vi "Init Airmar Serial.vi"(8 "error in (no error)":errorcluster, 10 "NotifierReff":T1, 11 "VISA Refnum in":refnum<visa-resource-name>="COM1") -> (0 "error out":errorcluster, 2 "Total number of connection attempts":i32, 3 "VISA Refnum out":refnum<visa-resource-name>)   [LabVIEW 2013]
doc: "This VI checks to see if the sensor is communicating on 4800 or 38400 baud and sets it to 38400 baud if it is not already."
uses:
  Data/TypeDefs/Notifiers.ctl
  Data/TypeDefs/UTM Location.ctl
  Data/TypeDefs/Sail Set Suggestions.ctl
  Data/TypeDefs/Rudder Set Suggestions.ctl
  Data/TypeDefs/OverrideInformation.ctl
  Data/TypeDefs/OverrideMode.ctl
  Data/TypeDefs/MotorSetup.ctl
  Data/TypeDefs/DynamixelSetupInfo.ctl
  Data/TypeDefs/AirmarStatus.ctl
  Data/TypeDefs/HardwareOnline.ctl
  Data/TypeDefs/DynamixelCycleTracker.ctl
  Data/TypeDefs/RC Input Values.ctl
  Classes/Waypoint/Waypoint.lvclass
panel:
  out "return count":u32
  out "read buffer 3":string
  out "read buffer 2":string
  out "read buffer":string
  out "# of 38400 baud attempts":i32
  out "# of 4800 baud attempts":i32
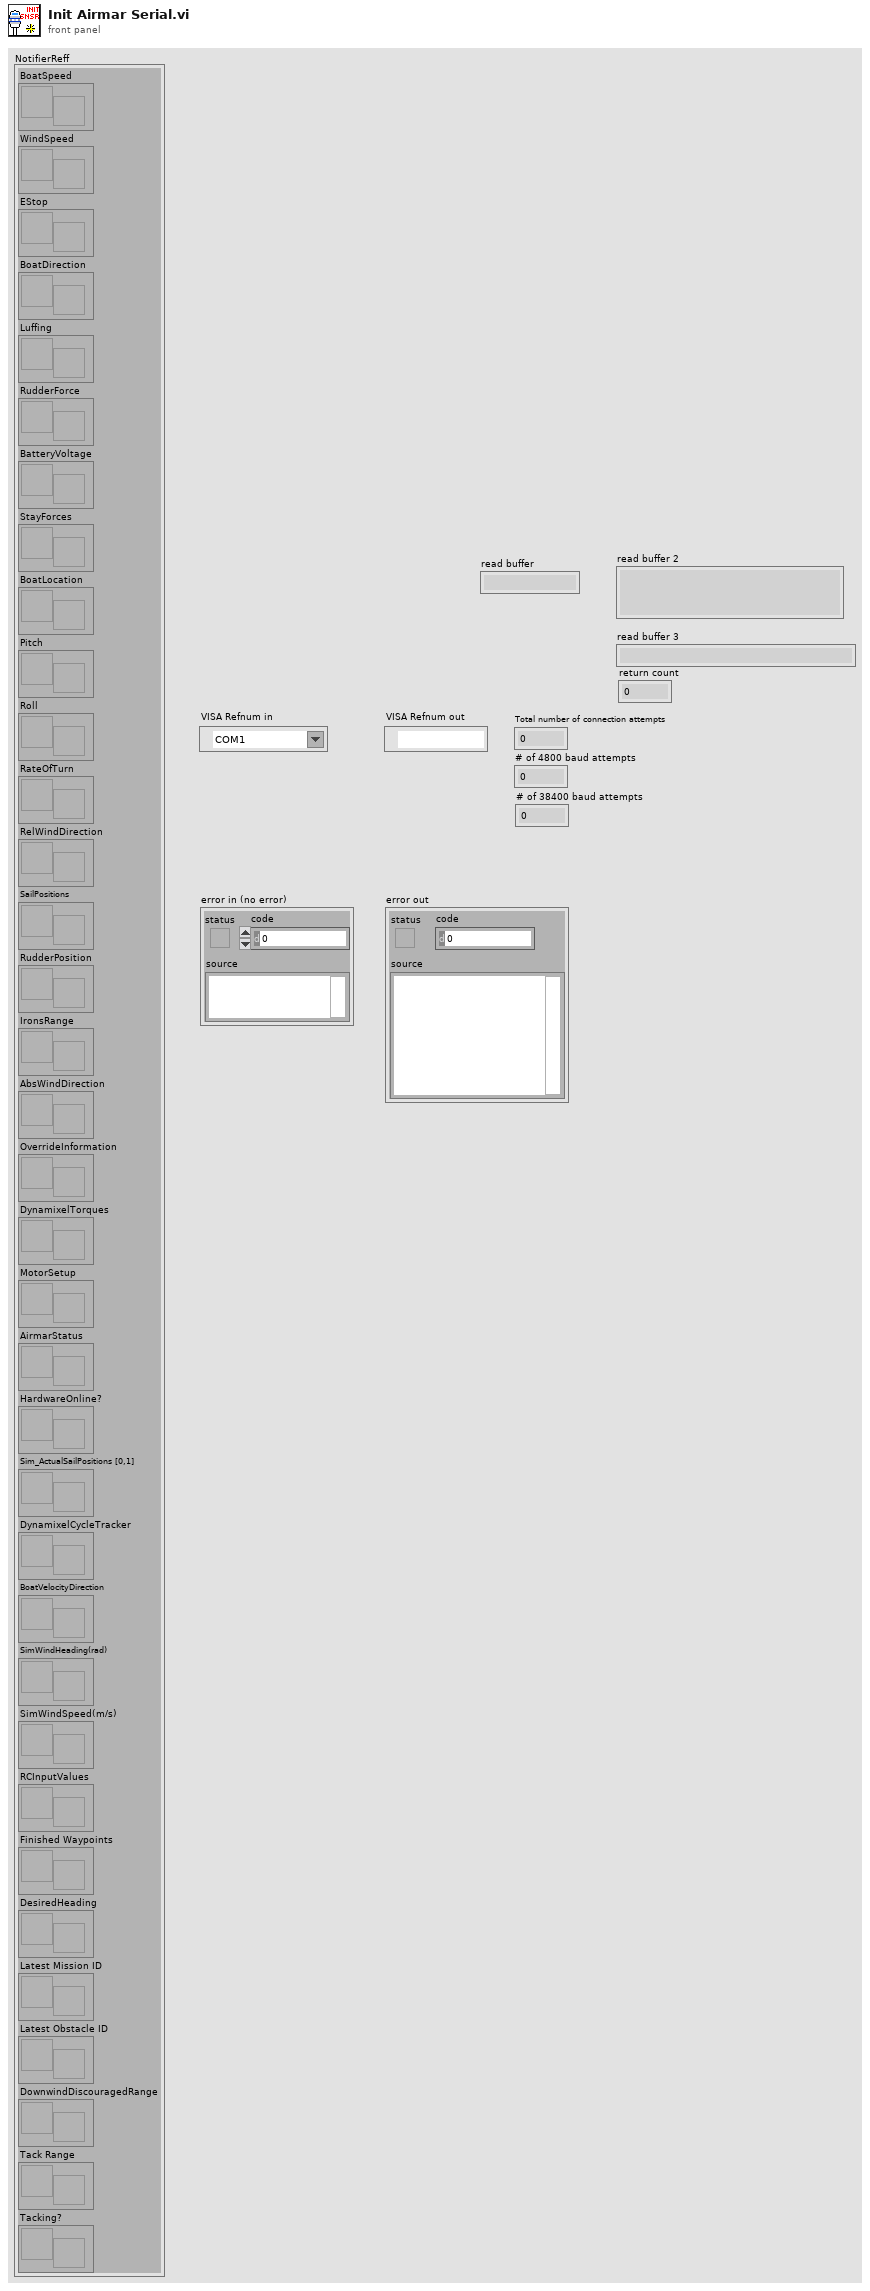
[diagram p1: front panel]
types:
  T1 = typedef "Notifiers.ctl" = cluster{"BoatSpeed":refnum<notifier>, "WindSpeed":refnum<notifier>, "EStop":refnum<notifier>, "BoatDirection":refnum<notifier>, "Luffing":refnum<notifier>, "RudderForce":refnum<notifier>, "BatteryVoltage":refnum<notifier>, "StayForces":refnum<notifier>, "BoatLocation":refnum<notifier>, "Pitch":refnum<notifier>, "Roll":refnum<notifier>, "RateOfTurn":refnum<notifier>, "RelWindDirection":refnum<notifier>, "SailPositions":refnum<notifier>, "RudderPosition":refnum<notifier>, "IronsRange":refnum<notifier>, "AbsWindDirection":refnum<notifier>, "OverrideInformation":refnum<notifier>, "DynamixelTorques":refnum<notifier>, "MotorSetup":refnum<notifier>, "AirmarStatus":refnum<notifier>, "HardwareOnline?":refnum<notifier>, "Sim_ActualSailPositions [0,1]":refnum<notifier>, "DynamixelCycleTracker":refnum<notifier>, "BoatVelocityDirection":refnum<notifier>, "SimWindHeading(rad)":refnum<notifier>, "SimWindSpeed(m/s)":refnum<notifier>, "RCInputValues":refnum<notifier>, "Finished Waypoints":refnum<notifier>, "DesiredHeading":refnum<notifier>, "Latest Mission ID":refnum<notifier>, "Latest Obstacle ID":refnum<notifier>, "DownwindDiscouragedRange":refnum<notifier>, "Tack Range":refnum<notifier>, "Tacking?":refnum<notifier>}
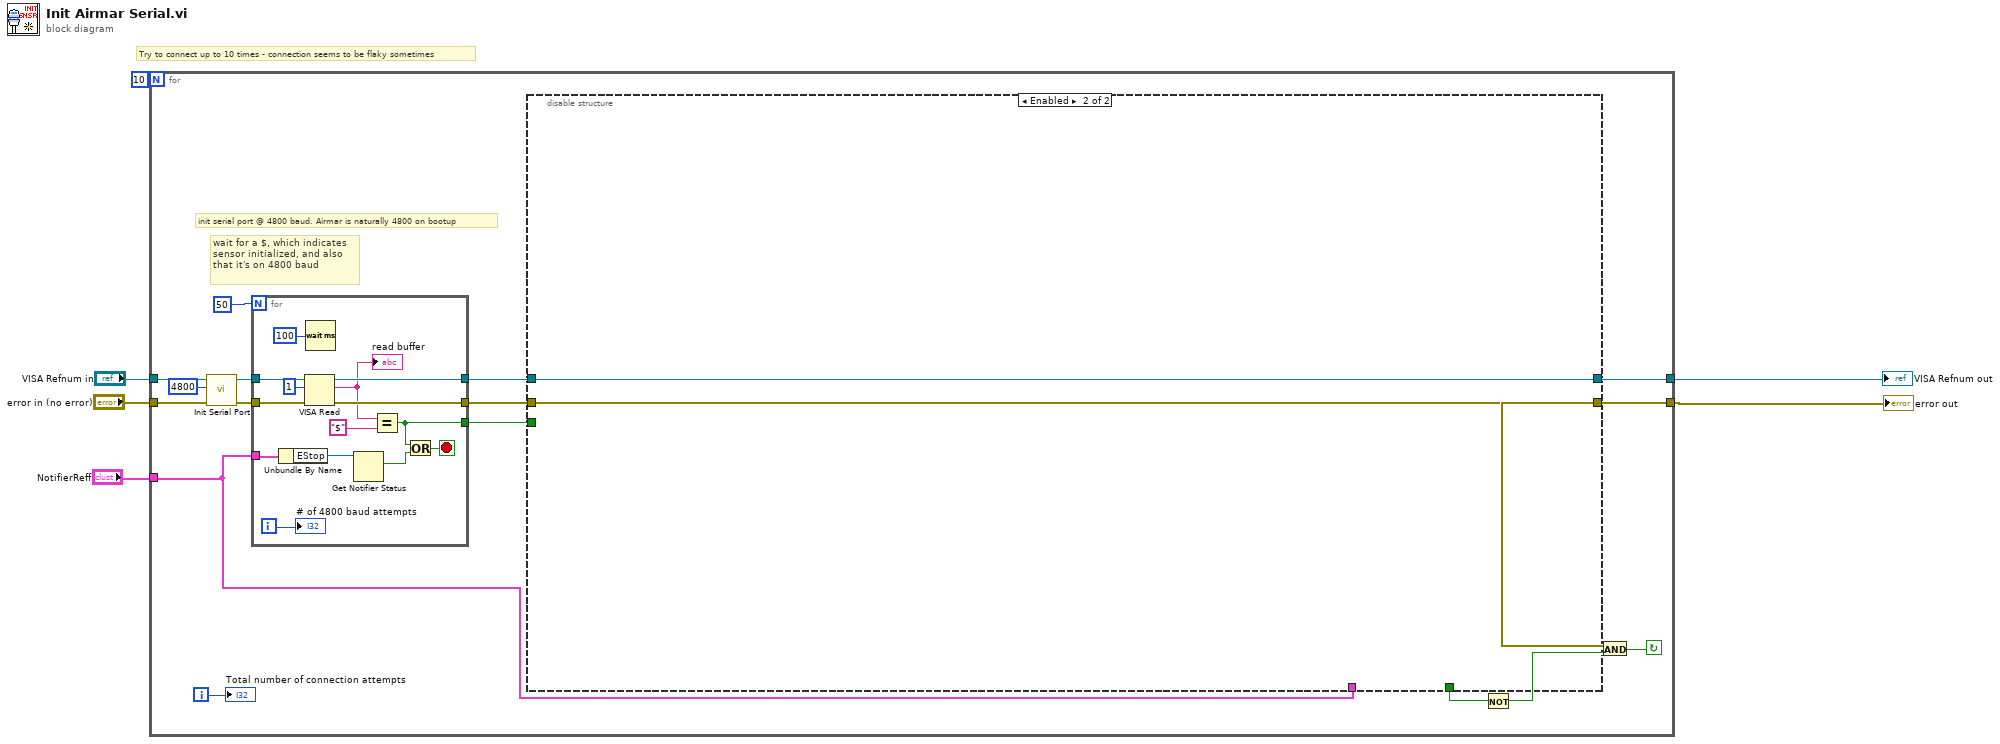
[diagram p0: block diagram]
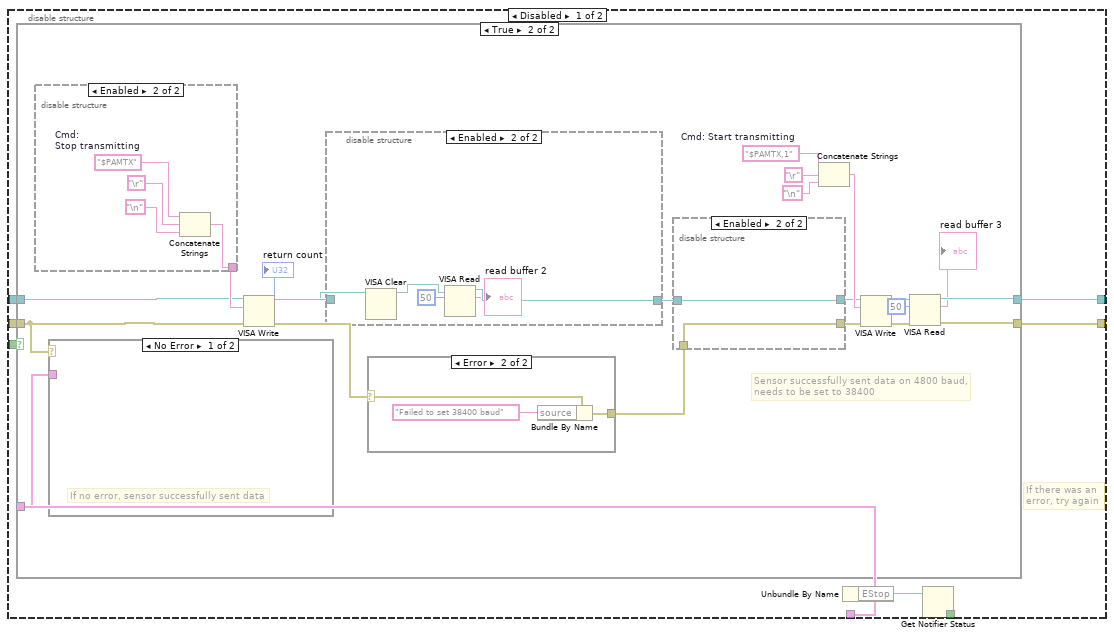
[diagram p2: hidden frame]
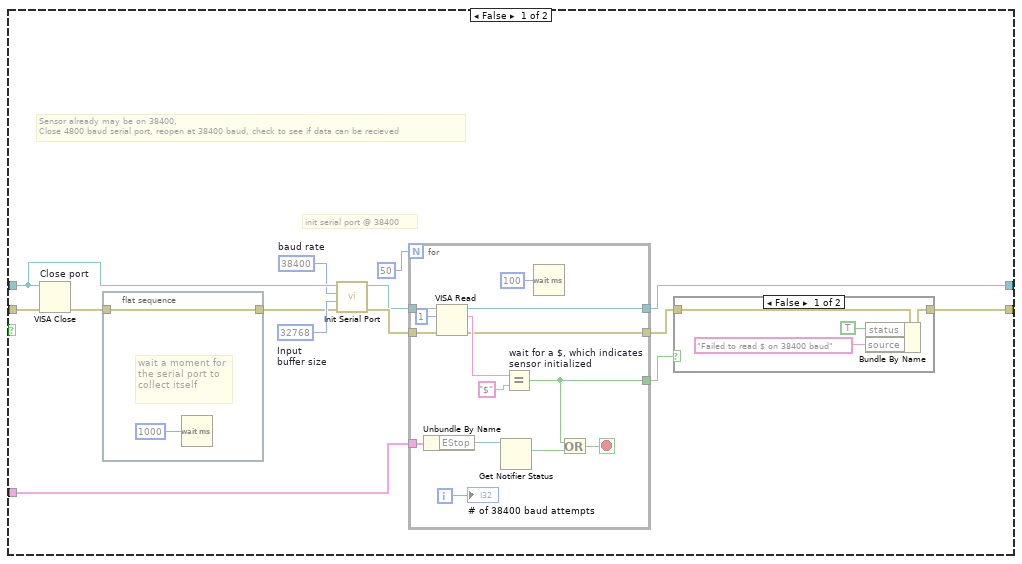
[diagram p3: hidden frame]
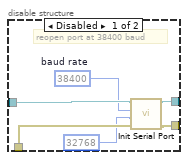
[diagram p5: hidden frame]
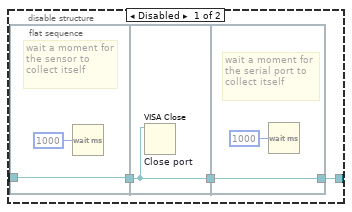
[diagram p6: hidden frame]
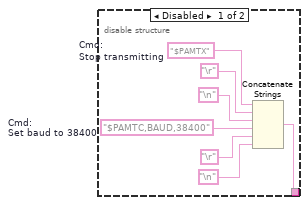
[diagram p7: hidden frame]
diagram:
  # "Try to connect up to 10 times - connection seems to be flaky sometimes"
  n1 = for {
    N: 10 -> [_]
    tunnel: "error in (no error)" -> [w12]
    tunnel: "VISA Refnum in" -> [w13]
    tunnel: [w22] -> w4
    tunnel: [w16] -> w3
    tunnel: "NotifierReff" -> [w8]
    i -> [w18]
    stop <- w17 continue-if-true
    # "wait for a $, which indicates sensor initialized, and also that it's on 4800 baud"
    # "init serial port @ 4800 baud. Airmar is naturally 4800 on bootup"
    n2 = call "Init Serial Port.vi"("error in (no error)"=w12, "baud rate"=u32 4800, "VISA Refnum in"=w13) -> ("error out"=w11:errorcluster, "VISA Refnum out"=w10:refnum<visa-resource-name>)  [unwired: 7 in]
    n3 = for {
      N: 50 -> [_]
      tunnel: [w139] -> w21
      tunnel: w10 -> [w138]
      tunnel: w11 -> [w137]
      tunnel: [w136] -> w20
      tunnel: [w131] -> w19
      tunnel: w8 -> [w129]
      i -> [w130]
      stop <- w132 stop-if-true
      n4 = Unbundle By Name(w129) -> ("EStop"=w128:refnum<notifier>)
      n5 = VISA Read(VISA resource name=w138, byte count=u32 1, error in (no error)=w137) -> (VISA resource name out=w139:refnum<visa-resource-name>, read buffer=w134:string, error out=w136:errorcluster)  [unwired: 1 out]
      "read buffer" <- w134
      n6 = Wait (ms)(milliseconds to wait=u32 100) -> ()  [unwired: 1 out]
      n7 = Get Notifier Status(notifier=w128) -> (current notification=w127:bool)  [unwired: 1 in, 4 out]
      n8 = Equal? ("wait for a $, which indicates\nsensor initialized")(x=w134, y="$" ("x")) -> (x = y?=w131:bool)
      n9 = Or(x=w131, y=w127) -> (x .or. y?=w132:bool)
      "# of 4800 baud attempts" <- w130
    }
    n10 = disable-structure shown="Enabled" {
      disable-tunnel: [w30 w125] -> w22
      disable-tunnel: w21 -> [w29 w125]
      disable-tunnel: w20 -> [w28 w124]
      disable-tunnel: w19 -> [w27 _]
      disable-tunnel: [w26 w124] -> w16
      disable-tunnel: [w25 _] -> w9
      disable-tunnel: w8 -> [w24 _]
      frame Disabled {
        # "If there was an \nerror, try again"
        n11 = case shown="True" w27 {
          tunnel: [w44 w73] -> w30
          tunnel: w29 -> [w37 w68]
          tunnel: w28 -> [w39 w67]
          tunnel: [w43 w72] -> w26
          tunnel: w24 -> [w31 w75]
          frame False {
            w35 = u32 32768  # Input buffer size
            w36 = u32 38400  # baud rate
            # "init serial port @ 38400"
            # "Sensor already may be on 38400,\nClose 4800 baud serial port, reopen at 38400 baud, check to see if data can be recieved"
            n12 = VISA Close "Close port"(VISA resource name=w37, error in (no error)=w39) -> (error out=w38:errorcluster)
            n13 = flat-sequence {
              tunnel: w38 -> [w45]
              tunnel: [w45] -> w34
              frame #0 {
                # "wait a moment for the serial port to collect itself"
                n14 = Wait (ms)(milliseconds to wait=u32 1000) -> ()  [unwired: 1 out]
              }
            }
            n15 = call "Init Serial Port.vi"("error in (no error)"=w34, "Input\nbuffer size"=w35, "baud rate"=w36, "VISA Refnum in"=w37) -> ("error out"=w33:errorcluster, "VISA Refnum out"=w32:refnum<visa-resource-name>)  [unwired: 6 in]
            n16 = for {
              N: 50 -> [_]
              tunnel: w32 -> [w60]
              tunnel: w33 -> [w59]
              tunnel: [w58] -> w44
              tunnel: [w52] -> w42
              tunnel: [w54] -> w41
              tunnel: w31 -> [w49]
              i -> [w51]
              stop <- w53 stop-if-true
              n17 = Unbundle By Name(w49) -> ("EStop"=w50:refnum<notifier>)
              n18 = VISA Read(VISA resource name=w60, byte count=u32 1, error in (no error)=w59) -> (VISA resource name out=w58:refnum<visa-resource-name>, read buffer=w56:string, error out=w54:errorcluster)  [unwired: 1 out]
              n19 = Get Notifier Status(notifier=w50) -> (current notification=w47:bool)  [unwired: 1 in, 4 out]
              n20 = Equal? "wait for a $, which indicates\nsensor initialized"(x=w56, y="$" ("x")) -> (x = y?=w52:bool)
              n21 = Wait (ms)(milliseconds to wait=u32 100) -> ()  [unwired: 1 out]
              n22 = Or(x=w52, y=w47) -> (x .or. y?=w53:bool)
              "# of 38400 baud attempts" <- w51
            }
            n23 = case shown="False" w42 {
              tunnel: w41 -> [w62 w65]
              tunnel: [w61 w65] -> w43
              frame False {
                n24 = Bundle By Name(cluster=w62, "status"=TRUE, "source"="Failed to read $ on 38400 baud") -> (w61:errorcluster)
              }
              frame True {
              }
            }
          }
          frame True {
            w86 = "$PAMTX,1"  # Cmd: Start transmitting
            # "Sensor successfully sent data on 4800 baud,\nneeds to be set to 38400"
            n25 = disable-structure shown="Enabled" {
              disable-tunnel: [w114 w116] -> w82
              frame Disabled {
                w111 = "$PAMTC,BAUD,38400"  # Cmd: Set baud to 38400
                w115 = "$PAMTX"  # Cmd: Stop transmitting
                n26 = Concatenate Strings(w115, "\r" ("Carriage Return Constant"), "\n", w111, "\r" ("Carriage Return Constant"), "\n") -> (w114:string)
              }
              frame Enabled {
                w119 = "$PAMTX"  # Cmd: Stop transmitting
                n27 = Concatenate Strings(w119, "\r" ("Carriage Return Constant"), "\n") -> (w116:string)
              }
            }
            n28 = case shown="No Error" w67 {
              tunnel: w75 -> [_ _]
              frame No Error {
                # "If no error, sensor successfully sent data"
              }
              frame Error {
              }
            }
            n29 = VISA Write(VISA resource name=w68, write buffer=w82, error in (no error)=w67) -> (VISA resource name out=w81:refnum<visa-resource-name>, return count=→"return count":u32, error out=w80:errorcluster)
            n30 = disable-structure shown="Enabled" {
              disable-tunnel: w81 -> [w96 w105]
              disable-tunnel: [w95 w108] -> w79
              frame Disabled {
                n31 = flat-sequence {
                  tunnel: w96 -> [w99]
                  tunnel: [w99] -> w98
                  tunnel: w98 -> [w101]
                  tunnel: [w101] -> w97
                  tunnel: [w103] -> w95
                  tunnel: w97 -> [w103]
                  frame #0 {
                    # "wait a moment for the sensor to collect itself"
                    n32 = Wait (ms)(milliseconds to wait=u32 1000) -> ()  [unwired: 1 out]
                  }
                  frame #1 {
                    n33 = VISA Close "Close port"(VISA resource name=w101) -> ()  [unwired: 1 in, 1 out]
                  }
                  frame #2 {
                    # "wait a moment for the serial port to collect itself"
                    n34 = Wait (ms)(milliseconds to wait=u32 1000) -> ()  [unwired: 1 out]
                  }
                }
              }
              frame Enabled {
                n35 = VISA Clear(VISA resource name=w105) -> (VISA resource name out=w104:refnum<visa-resource-name>)  [unwired: 1 in, 1 out]
                n36 = VISA Read(VISA resource name=w104, byte count=u32 50) -> (VISA resource name out=w108:refnum<visa-resource-name>, read buffer=→"read buffer 2":string)  [unwired: 1 in, 2 out]
              }
            }
            n37 = case shown="Error" w80 {
              selector: w80 -> [w120 w123]
              tunnel: [w120 w121] -> w76
              frame No Error {
              }
              frame Error {
                n38 = Bundle By Name(cluster=w123, "source"="Failed to set 38400 baud") -> (w121:errorcluster)
              }
            }
            n39 = disable-structure shown="Enabled" {
              disable-tunnel: w79 -> [w92 w94]
              disable-tunnel: [w91 w94] -> w78
              disable-tunnel: [w90 w93] -> w77
              disable-tunnel: w76 -> [w89 w93]
              frame Disabled {
                w87 = u32 38400  # baud rate
                # "reopen port at 38400 baud"
                n40 = call "Init Serial Port.vi"("error in (no error)"=w89, "Input\nbuffer size"=u32 32768 ("Input\nbuffer size"), "baud rate"=w87, "VISA Refnum in"=w92) -> ("error out"=w90:errorcluster, "VISA Refnum out"=w91:refnum<visa-resource-name>)  [unwired: 6 in]
              }
              frame Enabled {
              }
            }
            n41 = Concatenate Strings(w86, "\r" ("Carriage Return Constant"), "\n") -> (w83:string)
            n42 = VISA Write(VISA resource name=w78, write buffer=w83, error in (no error)=w77) -> (VISA resource name out=w74:refnum<visa-resource-name>, error out=w71:errorcluster)  [unwired: 1 out]
            n43 = VISA Read(VISA resource name=w74, byte count=u32 50, error in (no error)=w71) -> (VISA resource name out=w73:refnum<visa-resource-name>, read buffer=→"read buffer 3":string, error out=w72:errorcluster)  [unwired: 1 out]
          }
        }
        n44 = Unbundle By Name(w24) -> ("EStop"=w23:refnum<notifier>)
        n45 = Get Notifier Status(notifier=w23) -> (current notification=w25:bool)  [unwired: 1 in, 4 out]
      }
      frame Enabled {
      }
    }
    n46 = Not(x=w9) -> (.not. x?=w15:bool)
    n47 = And(x=w16, y=w15) -> (x .and. y?=w17:bool)
    "Total number of connection attempts" <- w18
  }
  "VISA Refnum out" <- w4
  "error out" <- w3
